vi "例程10-使用定时循环生产波形.vi"() -> ()   [LabVIEW 2016]
uses:
  <vilib>/Platform/TimedLoop/XDataNode/timing_clust.ctl
  <vilib>/Platform/TimedLoop/XDataNode/nitl_modes.ctl
  <vilib>/Platform/TimedLoop/XDataNode/wakeup.ctl
  <vilib>/Platform/TimedLoop/XDataNode/XDataNode.xnode
  <vilib>/Platform/TimedLoop/XDataNode/XDNodeRunTimeDep.lvlib
panel:
  out "添加的数组":i64[][](array[numeric])
  out "波形图":i64[][](graph)
  in  "偏移量 2":i64
  in  "周期 2":i64
  in  "输入数":i64
  in  "周期":i64
  in  "偏移量":i64
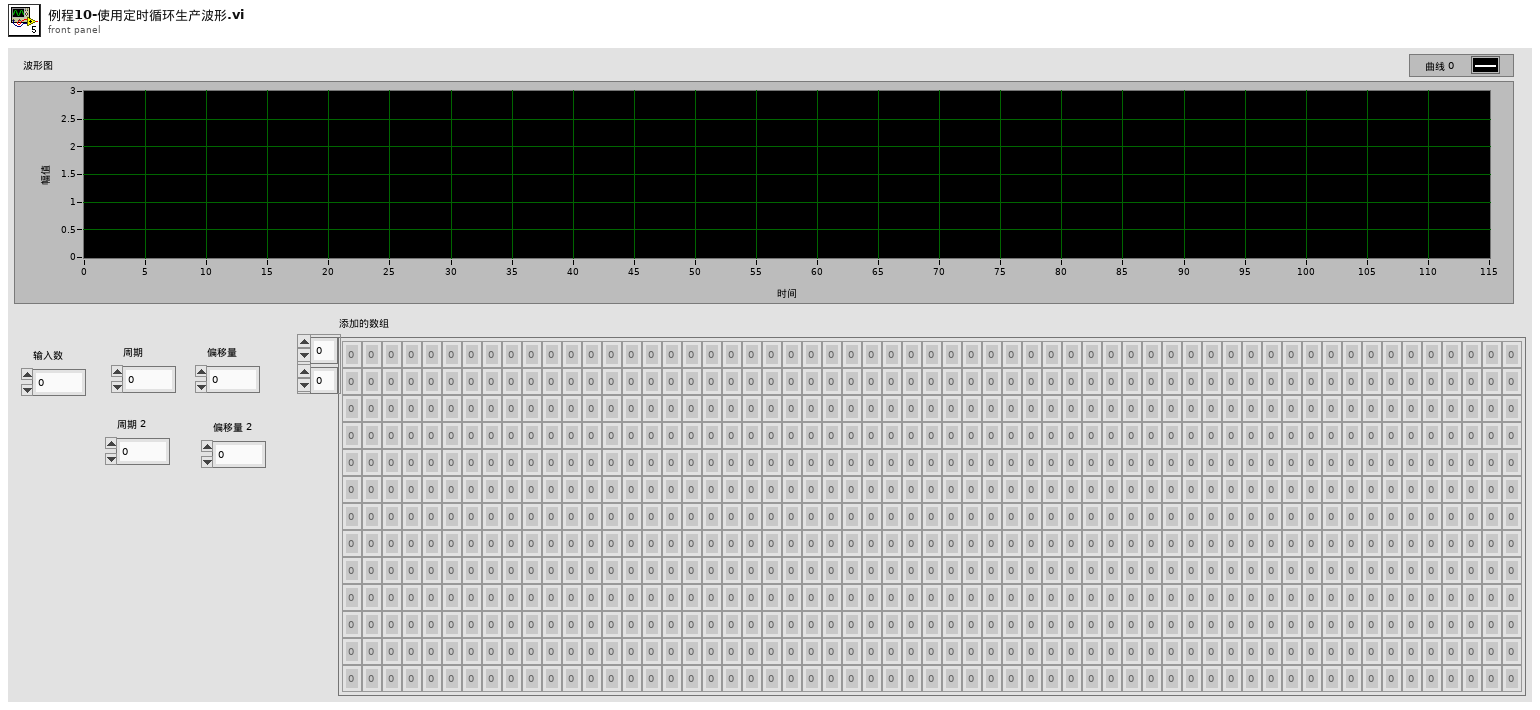
[diagram p1: front panel]
types:
  T1 = typedef "XDNodeRunTimeDep.lvlib/timing_clust.ctl" = cluster{"Expected End [f-1]":u64, "Actual End [f-1]":u64, "Finished Late? [f-1]":bool, "Expected End [i-1]":u64, "Actual End [i-1]":u64, "Finished Late? [i-1]":bool, "Expected Start [i]":u64, "Actual Start [i]":u64, "Expected Start [f]":u64, "Actual Start [f]":u64, "Source Name":string, "Structure Name":string, "Period":i64, "Deadline":i64, "Offset":i64, "Start":i64, "Priority":i32, "Timeout":i32, "Mode":T2, "Wakeup Reason":T3, "Error":errorcluster, "Source Type":string, "Secondary Source Type":string, "Global End Time":u64, "Global Start Time":u64, "Frame Duration":u64, "Iteration Duration":u64, "Assigned CPU":i32, "I/O Scan Engine Mode":u32}
  T2 = typedef "XDNodeRunTimeDep.lvlib/nitl_modes.ctl" = enum32{"No Change", "Process missed periods, maintain original phase", "Discard missed periods, maintain original phase", "Process missed periods, ignore original phase", "Discard missed periods, ignore original phase"}
  T3 = typedef "XDNodeRunTimeDep.lvlib/wakeup.ctl" = enum32{"Normal", "Aborted", "Asynchronous wakeup", "Timing source error", "Timed loop error", "Timeout"}
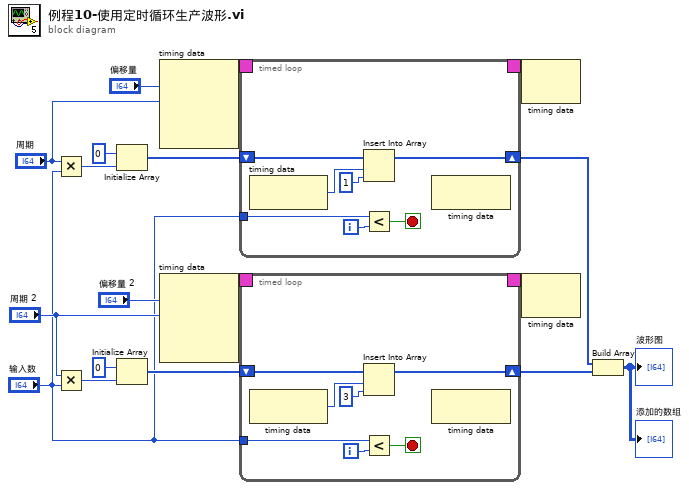
[diagram p0: block diagram]
diagram:
  n1 = Multiply(x="周期", y="输入数") -> (x*y=w12:i64)
  n2 = Multiply(x="周期 2", y="输入数") -> (x*y=w7:i64)
  n3 = Initialize Array(i64 0 ("元素"), w12) -> (w14:i64[])
  n4 = Initialize Array(i64 0 ("元素"), w7) -> (w5:i64[])
  n5 = node-c288("偏移量", "周期") -> (w18:T1)  [unwired: 2 in]
  n6 = node-c288("偏移量 2", "周期 2") -> (w16:T1)  [unwired: 2 in]
  n7 = timed-loop {
    timing: w18 -> [_]
    timing-out: [_] -> w17
    tunnel: "输入数" -> [w23]
    shift-right: [w19] -> w4
    shift-left: w14 -> [w21]
    i -> [w25]
    stop <- w24 stop-if-true
    n8 = node-c288() -> (w22:i64)  [unwired: 1 in]
    n9 = Insert Into Array(array=w21, index=w22, new element=i64 1 ("新元素/子数组")) -> (w19:i64[])
    n10 = Less?(x=w23, y=w25) -> (x < y?=w24:bool)
    n11 = node-c288() -> ()  [unwired: 1 in, 1 out]
  }
  n12 = timed-loop {
    timing: w16 -> [_]
    timing-out: [_] -> w15
    tunnel: "输入数" -> [w30]
    shift-right: [w29] -> w2
    shift-left: w5 -> [w32]
    i -> [w35]
    stop <- w34 stop-if-true
    n13 = node-c288() -> (w33:i64)  [unwired: 1 in]
    n14 = Insert Into Array(array=w32, index=w33, new element=i64 3 ("新元素/子数组")) -> (w29:i64[])
    n15 = Less?(x=w30, y=w35) -> (x < y?=w34:bool)
    n16 = node-c288() -> ()  [unwired: 1 in, 1 out]
  }
  n17 = node-c288(w17) -> ()  [unwired: 1 out]
  n18 = node-c288(w15) -> ()  [unwired: 1 out]
  n19 = Build Array(w4, w2) -> (→"波形图" →"添加的数组":i64[][])
